vi "多参数断电保存全局变量.vi"() -> ()   [LabVIEW 2016, in "斯坦道仪器.lvlib"]
panel:
  in  "质控参数设置":T1
  # "质控参数设置"
  # "监测参数"
  # "水温"
  # "酸碱度"
  # "溶解氧"
  # "电导率"
  # "浊度"
  # "标样核查标准液浓度"
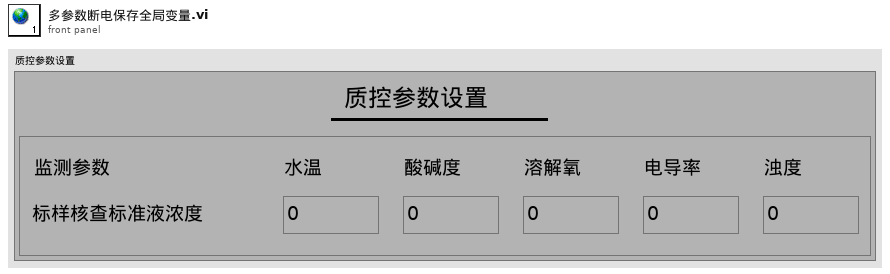
[diagram p1: front panel]
types:
  T1 = cluster{"水温标准液标准浓度":dbl, "酸碱度标准液标准浓度":dbl, "溶解氧标准液标准浓度":dbl, "电导率标准液标准浓度":dbl, "浊度标准液标准浓度":dbl}
diagram:
